vi "Build Create.vi"(8 "error in (no error)":errorcluster, 9 "tableName":string, 10 "DynamicParameters in":refnum<class "DynamicParameters.lvclass">, 11 "KDBConnection in":refnum<class "DBC.lvclass">) -> (0 "error out":errorcluster, 1 "LastIdentityQuery":string, 2 "InsertStatement":string, 3 "KDBConnection out":refnum<class "DBC.lvclass">)   [LabVIEW 2020, in "ORM_DBC_Kdb.lvlib" / "DBC.lvclass"]
uses:
  DBC.lvclass
  C:/Program Files (x86)/National Instruments/LabVIEW 2020/vi.lib/Viviota/shared/ORM.lvlibp/ORM/DbConnection/DbConnection.lvclass
  <vilib>/Viviota/shared/ORM.lvlibp/ORM/DynamicParameters/DynamicParameters.lvclass
  <vilib>/Viviota/shared/ORM.lvlibp/ORM/DynamicParameters/Read ParameterNames.vi
  <vilib>/Viviota/shared/ORM.lvlibp/ORM/DynamicParameters/Read FieldNames.vi
  <vilib>/Viviota/shared/ORM.lvlibp/ORM/DbConnection/Read LastIdentityQuery.vi
  <vilib>/Viviota/shared/ORM.lvlibp/ORM/DbConnection/Read ColumnNameFormat.vi
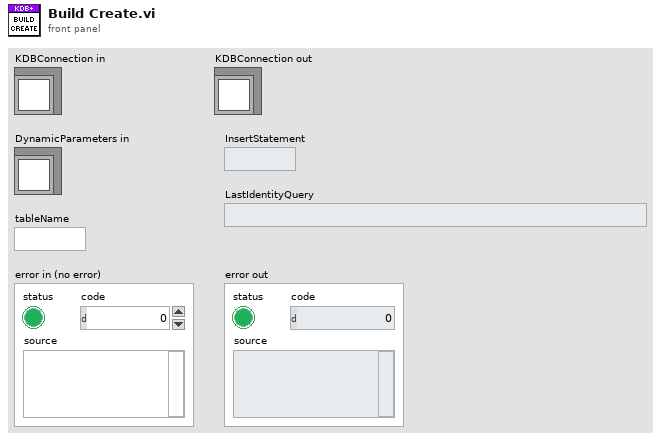
[diagram p1: front panel]
types:
  T1 = typedef "ORM_DBC_Kdb.lvlib/DBC.lvclass/kdb_TableType_enum.ctl" = enum16{"Memory", "Disk_Serialized", "Disk_Splayed", "Disk_Partitioned", "Other"}
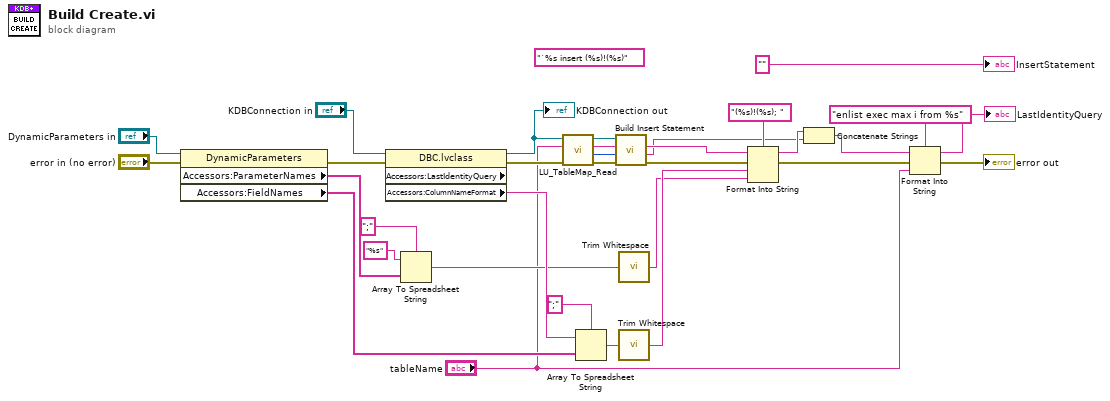
[diagram p0: block diagram]
diagram:
  (unwired) "`%s insert (%s)!(%s)"
  n1 = property class="DynamicParameters"(reference="DynamicParameters in", error in="error in (no error)") -> (error out=w17:errorcluster, "Accessors:ParameterNames"=w27:string[], "Accessors:FieldNames"=w31:string[])  [unwired: 1 out]
  n2 = property class="DBC.lvclass" props=["Accessors:LastIdentityQuery", "Accessors:ColumnNameFormat"](reference="KDBConnection in", error in=w17) -> (reference out=w14:refnum<class "DBC.lvclass">, error out=w15:errorcluster, "Accessors:ColumnNameFormat"=w26:string)  [unwired: 1 out]
  "KDBConnection out" <- w14
  n3 = Array To Spreadsheet String(delimiter (Tab)=";", array=w27, 3:"%s" ("format string")) -> (spreadsheet string=w24:string)
  n4 = call "LU_TableMap_Read.vi"("error in (no error)"=w15, "TableName"="tableName", "KDBConnection in"=w14) -> ("error out"=w12:errorcluster, "TableType"=w11:T1, "TableName Out"=w10:string, "KDBConnection out"=w9:refnum<class "DBC.lvclass">)  [unwired: 5 in]
  n5 = Array To Spreadsheet String(delimiter (Tab)=";", array=w31, 3:w26) -> (spreadsheet string=w29:string)
  n6 = call "Build Insert Statement.vi"("error in (no error)"=w12, "TableType"=w11, "TableName"=w10, "KDBConnection in"=w9) -> ("error out"=w7:errorcluster, "Insert Statement Suffix"=w3:string, "Initial Insert Statement Prefix"=w8:string)  [unwired: 4 in, 1 out]
  n7 = call <vilib>:"Trim Whitespace.vi"("string"=w24) -> ("trimmed string"=w25:string)  [unwired: 1 in]
  n8 = call <vilib>:"Trim Whitespace.vi"("string"=w29) -> ("trimmed string"=w28:string)  [unwired: 1 in]
  n9 = Format Into String(format string="(%s)!(%s); ", initial string=w8, error in=w7, w28, w25) -> (resulting string=w4:string, error out=→"error out":errorcluster)
  n10 = Concatenate Strings(w4, w3) -> (w2:string)
  n11 = Format Into String(format string="enlist exec max i from %s", initial string=w2, "tableName") -> (resulting string=→"LastIdentityQuery":string)  [unwired: 1 in, 1 out]
  "InsertStatement" <- "" ("LastIdentityQuery")
